vi "配置读取与写入.vi"(7 "功能":enum16{"读取", "写入"}(ring), 8 "error in (no error)":errorcluster, 11 "连接配置":T1={"连接类型"=enum."TCP", "串口"="COM3", "IP"="192.168.1.200", "PORT"=502}) -> (0 "error out":errorcluster, 3 "连接配置 2":T1={"连接类型"=enum."TCP", "串口"="COM3", "IP"="192.168.1.200", "PORT"=502})   [LabVIEW 2016, in "PLC.lvlib"]
uses:
  PLC.lvlib
  <vilib>/Utility/config.llb/NI_LVConfig.lvlib
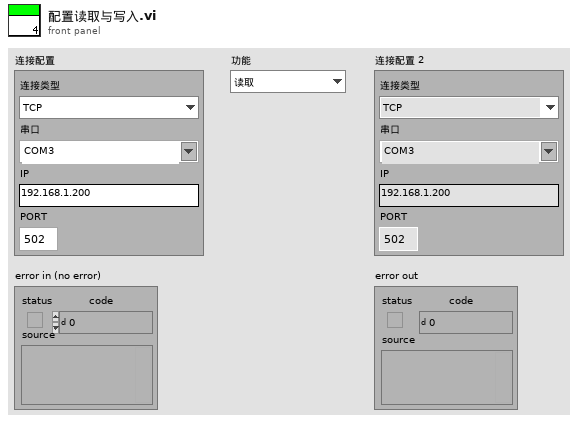
[diagram p1: front panel]
types:
  T1 = cluster{"连接类型":enum16{"串口", "TCP"}, "串口":string, "IP":string, "PORT":u16}
  T2 = typedef "NI_LVConfig.lvlib/Config Data RefNum.ctl" = refnum<k1>
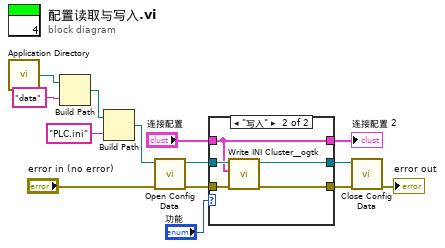
[diagram p0: block diagram]
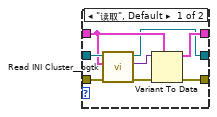
[diagram p2: hidden frame]
diagram:
  n1 = call <vilib>:"Application Directory.vi"() -> ("Application Directory"=w6:path)
  n2 = Build Path(base path=w6, name or relative path="data") -> (appended path=w4:path)
  n3 = Build Path(base path=w4, name or relative path="PLC.ini") -> (appended path=w2:path)
  n4 = call <vilib>:"Open Config Data.vi"("error in (no error)"="error in (no error)", "configuration file path"=w2) -> ("error out"=w11:errorcluster, "refnum"=w12:T2)  [unwired: 7 in, 1 out]
  n5 = case shown="\"写入\"" "功能" {
    tunnel: "连接配置" -> [w19 w23]
    tunnel: w12 -> [w22 w27]
    tunnel: w11 -> [w21 w26]
    tunnel: [w15 w25] -> w10
    tunnel: [w16 w24] -> w9
    tunnel: [w18 w23] -> w1
    frame "读取", Default {
      n6 = call <userlib>:"Read INI Cluster__ogtk.vi"("error in (no error)"=w21, "INI Fomatted Cluster Type"=w19, "refnum"=w22) -> ("error out"=w17:errorcluster, "INI Fomatted Cluster"=w20:variant, "dup refnum"=w15:T2)  [unwired: 4 in, 2 out]
      n7 = Variant To Data(error in=w17, type=w19, Variant=w20) -> (data=w18:T1, error out=w16:errorcluster)
    }
    frame "写入" {
      n8 = call <userlib>:"Write INI Cluster__ogtk.vi"("error in (no error)"=w26, "INI Fomatted Cluster"=w23, "refnum"=w27) -> ("error out"=w24:errorcluster, "dup refnum"=w25:T2)  [unwired: 7 in]
    }
  }
  "连接配置 2" <- w1
  n9 = call <vilib>:"Close Config Data.vi"("error in (no error)"=w9, "refnum"=w10) -> ("error out"=→"error out":errorcluster)  [unwired: 8 in, 1 out]
